vi "Launch.vi"(8 "error in (no error)":errorcluster, 10 "Run":bool, 11 "Library Instr in":refnum<class "Library Instr.lvclass">) -> (0 "error out":errorcluster, 3 "Library Instr out":refnum<class "Library Instr.lvclass">)   [LabVIEW 2015, in "Item Actor.lvlib" / "Library Instr.lvclass"]
uses:
  Library Instr.lvclass
  Instrument Information/Instrument.lvclass/Instrument.ctl
  Instrument Information/Read App Path.vi
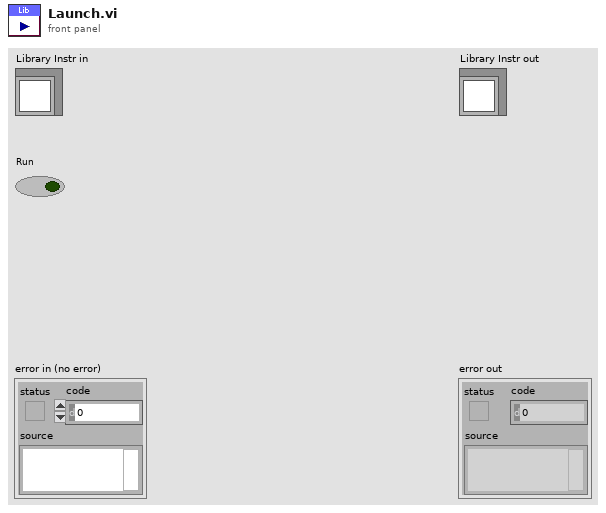
[diagram p1: front panel]
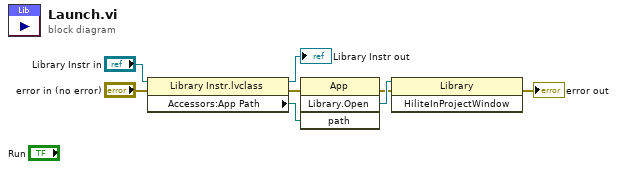
[diagram p0: block diagram]
diagram:
  n1 = property class="Library Instr.lvclass"(reference="Library Instr in", error in="error in (no error)") -> (reference out=→"Library Instr out":refnum<class "Library Instr.lvclass">, error out=w5:errorcluster, "Accessors:App Path"=w6:path)
  n2 = invoke class="App" method="Library.Open"(error in=w5, "path"=w6) -> (error out=w2:errorcluster, "Open Library"=w3:refnum<vi>)  [unwired: 2 in, 2 out]
  n3 = invoke class="Library" method="HiliteInProjectWindow"(reference=w3, error in=w2) -> (error out=→"error out":errorcluster)  [unwired: 1 in, 2 out]
